vi "Subtract.vi"(8 "error in (no error)":errorcluster, 10 "High Res Arithmetic 2":refnum<class "High Res Arithmetic.lvclass">, 11 "High Res Arithmetic 1":refnum<class "High Res Arithmetic.lvclass">) -> (0 "error out":errorcluster, 3 "High Res Arithmetic sum":refnum<class "High Res Arithmetic.lvclass">)   [LabVIEW 2021, in "High Res Arithmetic.lvclass"]
uses:
  High Res Arithmetic.lvclass
  High Res Arithmetic.lvclass/High Res Arithmetic.ctl
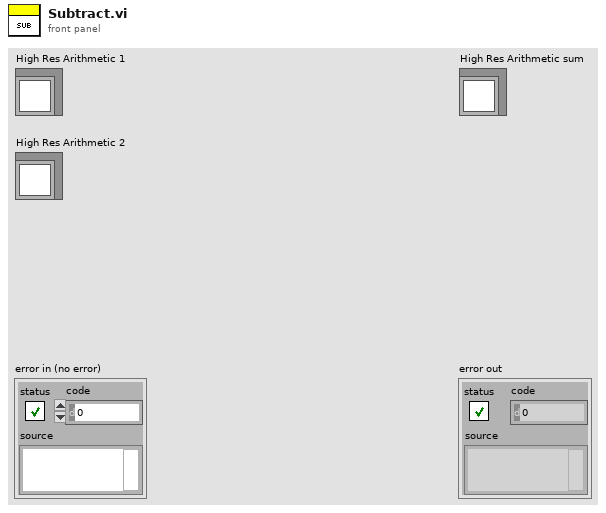
[diagram p1: front panel]
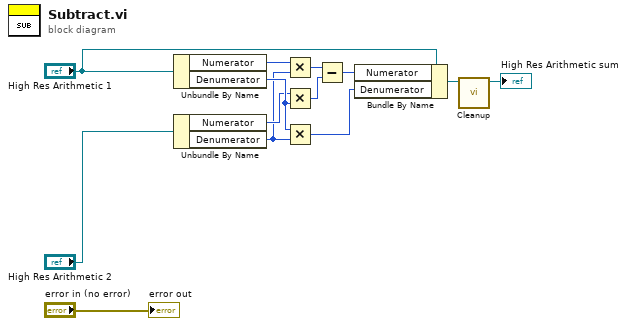
[diagram p0: block diagram]
diagram:
  n1 = Unbundle By Name("High Res Arithmetic 1") -> ("Numerator"=w3:i64, "Denumerator"=w6:i64)
  n2 = Unbundle By Name("High Res Arithmetic 2") -> ("Numerator"=w5:i64, "Denumerator"=w4:i64)
  n3 = Multiply(x=w3, y=w4) -> (x*y=w7:i64)
  n4 = Multiply(x=w5, y=w6) -> (x*y=w8:i64)
  n5 = Multiply(x=w6, y=w4) -> (x*y=w10:i64)
  n6 = Subtract(x=w7, y=w8) -> (x-y=w9:i64)
  n7 = Bundle By Name(cluster="High Res Arithmetic 1", "Numerator"=w9, "Denumerator"=w10) -> (w11:refnum<class "High Res Arithmetic.lvclass">)
  n8 = call "Cleanup.vi"("High Res Arithmetic in"=w11) -> ("High Res Arithmetic out"=→"High Res Arithmetic sum":refnum<class "High Res Arithmetic.lvclass">)  [unwired: 9 in, 1 out]
  "error out" <- "error in (no error)"
